vi "dump.vi"(8 "error in (no error)":errorcluster, 10 "indent":T1, 11 "FunctionType in":refnum<class "FunctionType.lvclass">) -> (0 "error out":errorcluster, 2 "mlir":string, 3 "FunctionType out":refnum<class "FunctionType.lvclass">)   [LabVIEW 2020, in "mlir.lvlib" / "FunctionType.lvclass"]
uses:
  FunctionType.lvclass
  Node/indent.ctl
  FunctionType.lvclass/FunctionType.ctl
  a1082ed8-b279-4973-ac16-a283b3d2b7e9.vi
  75b1669a-7995-4cea-925e-e7488a8fc09f.vi
  360a1896-477e-4c5d-9505-69496679b0e9.vi
  a1082ed8-b279-4973-ac16-a283b3d2b7e9.vi/2912b9a7-86c0-42e6-9e11-6b326dc4d0bc.vi
  75b1669a-7995-4cea-925e-e7488a8fc09f.vi/2912b9a7-86c0-42e6-9e11-6b326dc4d0bc.vi
  360a1896-477e-4c5d-9505-69496679b0e9.vi/2912b9a7-86c0-42e6-9e11-6b326dc4d0bc.vi
  Type/Type.lvclass
  Y:/FlowRails/mlir-labview/mlir-labview/Node/Node.lvclass
  _dump_or_value.vi
  Node/Node.lvclass
  mlir.lvlib
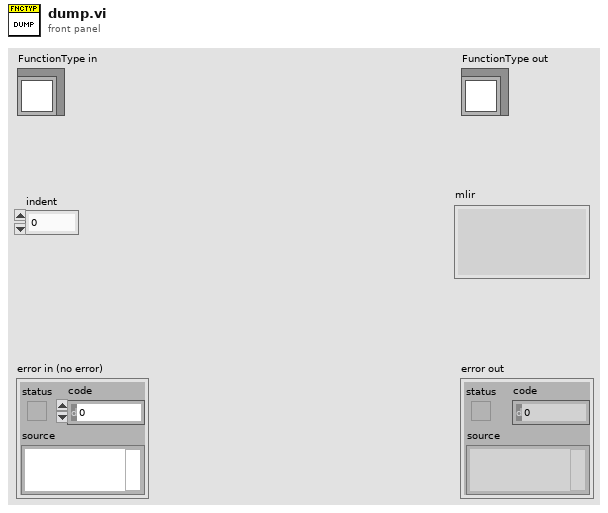
[diagram p1: front panel]
types:
  T1 = typedef "mlir.lvlib/indent.ctl" = u32
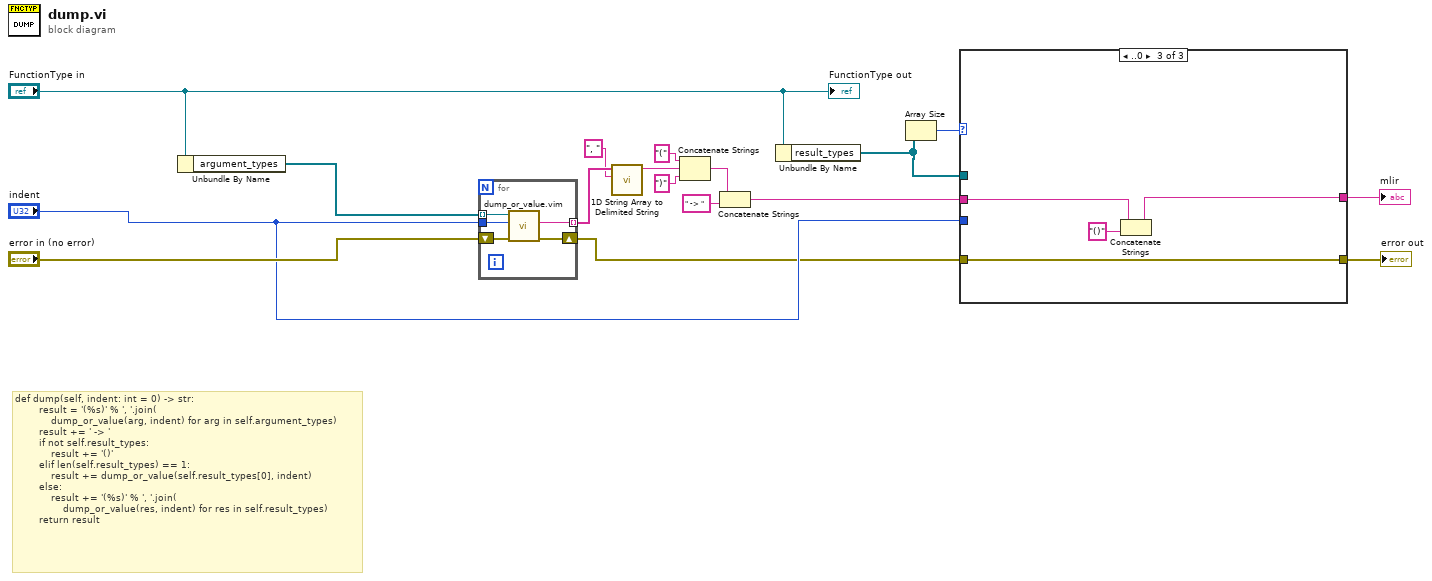
[diagram p0: block diagram]
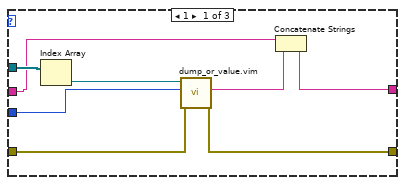
[diagram p2: hidden frame]
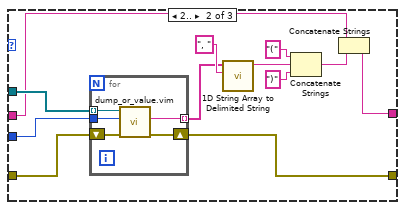
[diagram p3: hidden frame]
diagram:
  # "def dump(self, indent: int = 0) -> str:\n        result = '(%s)' % ', '.join(\n            dump_or_value(arg, indent) for arg in self.argument_types)\n        result += ' -> '\n        if not self.result_types:\n            result += '()'\n        elif len(self.result_types) == 1:\n            result += dump_or_value(self.result_types[0], indent)\n        else:\n            result += '(%s)' % ', '.join(\n                dump_or_value(res, indent) for res in self.result_types)\n        return result"
  n1 = Unbundle By Name("FunctionType in") -> ("argument_types"=w17:refnum<class "Type.lvclass">[])
  n2 = for {
    tunnel: w17 -> [w22] mode=indexing
    tunnel: "indent" -> [w21]
    shift-right: [w20] -> w2
    shift-left: "error in (no error)" -> [w19]
    tunnel: [w18] -> w15 mode=indexing
    n3 = call "dump_or_value.vim"("error in (no error)"=w19, "indent"=w21, "value"=w22) -> ("error out"=w20:errorcluster, "mlir"=w18:string)  [unwired: 7 in]
  }
  n4 = call <vilib>:"1D String Array to Delimited String.vi"("delimiter"=", ", "string array"=w15) -> ("delimited string"=w13:string)  [unwired: 9 in]
  n5 = Concatenate Strings("(" ("string"), w13, ")" ("string")) -> (w9:string)
  n6 = Concatenate Strings(w9, " -> " ("string")) -> (w7:string)
  n7 = Unbundle By Name("FunctionType in") -> ("result_types"=w5:refnum<class "Type.lvclass">[])
  n8 = Array Size(array=w5) -> (size(s)=w4:i32)
  n9 = case shown="..0" w4 {
    tunnel: w7 -> [w25 w33 w51]
    tunnel: w5 -> [w30 w37 _]
    tunnel: [w23 w32 w49] -> w6
    tunnel: "indent" -> [w28 w35 _]
    tunnel: w2 -> [w27 w36 w48]
    tunnel: [w26 w31 w48] -> w1
    frame 1 {
      n10 = Index Array(array=w30) -> (element=w29:refnum<class "Type.lvclass">)  [unwired: 1 in]
      n11 = call "dump_or_value.vim"("error in (no error)"=w27, "indent"=w28, "value"=w29) -> ("error out"=w26:errorcluster, "mlir"=w24:string)  [unwired: 7 in]
      n12 = Concatenate Strings(w25, w24) -> (w23:string)
    }
    frame 2.. {
      n13 = for {
        tunnel: w37 -> [w47] mode=indexing
        tunnel: w35 -> [w46]
        shift-right: [w45] -> w31
        shift-left: w36 -> [w44]
        tunnel: [w43] -> w38 mode=indexing
        n14 = call "dump_or_value.vim"("error in (no error)"=w44, "indent"=w46, "value"=w47) -> ("error out"=w45:errorcluster, "mlir"=w43:string)  [unwired: 7 in]
      }
      n15 = call <vilib>:"1D String Array to Delimited String.vi"("delimiter"=", ", "string array"=w38) -> ("delimited string"=w40:string)  [unwired: 9 in]
      n16 = Concatenate Strings("(" ("string"), w40, ")" ("string")) -> (w34:string)
      n17 = Concatenate Strings(w33, w34) -> (w32:string)
    }
    frame ..0 {
      n18 = Concatenate Strings(w51, "()" ("string")) -> (w49:string)
    }
  }
  "error out" <- w1
  "mlir" <- w6
  "FunctionType out" <- "FunctionType in"
